vi "arrayMax.vi"(11 "Array":dbl[](array[numeric])) -> (3 "Maxed array":dbl[](array[numeric]))   [LabVIEW 2012]
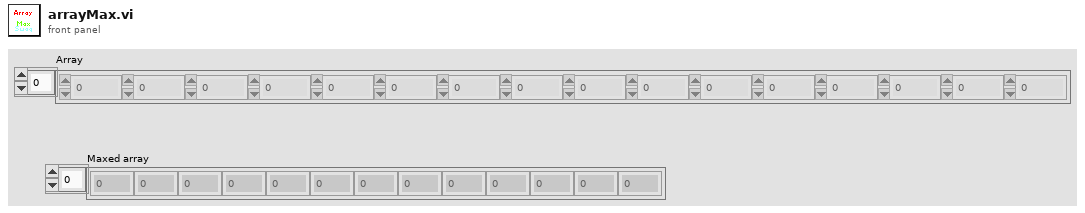
[diagram p1: front panel]
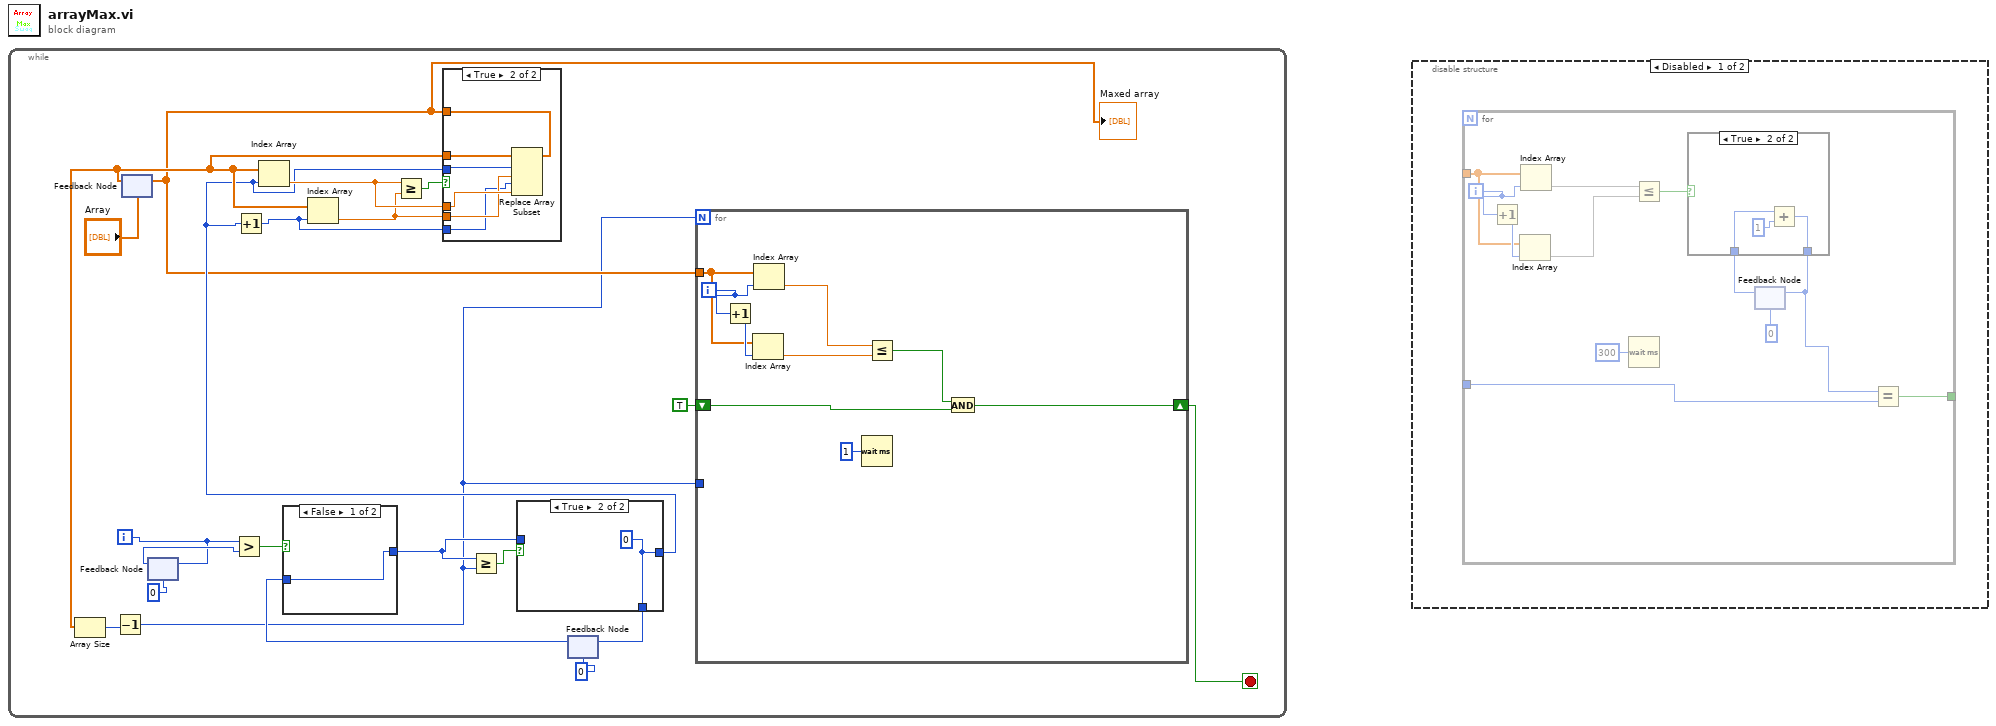
[diagram p0: block diagram]
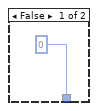
[diagram p2: hidden frame]
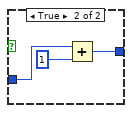
[diagram p5: hidden frame]
diagram:
  n1 = while {
    i -> [w18]
    stop <- w1 stop-if-true
    n2 = feedback #1("Array") -> (w10:dbl[])
    n3 = Array Size(array=w10) -> (size(s)=w4:i32)
    n4 = Decrement(x=w4) -> (x-1=w3:i32)
    n5 = feedback-in #2(w18) -> ()
    n6 = feedback #2(0) -> (w19:i32)
    n7 = Greater?(x=w18, y=w19) -> (0:w17:bool)
    n8 = feedback #3(0) -> (w8:i32)
    n9 = case shown="False" w17 {
      tunnel: [w33 w36] -> w15
      tunnel: w8 -> [w33 w34]
      frame False {
      }
      frame True {
        n10 = Add(x=w34, y=1) -> (x+y=w36:i32)
      }
    }
    n11 = Greater Or Equal?(x=w15, y=w3) -> (x >= y?=w16:bool)
    n12 = case shown="True" w16 {
      tunnel: [w31 w32] -> w6
      tunnel: w15 -> [w31 _]
      tunnel: [w31 w32] -> w7
      frame False {
      }
      frame True {
        w32 = 0
      }
    }
    n13 = Increment(x=w6) -> (x+1=w14:i32)
    n14 = Index Array(array=w10, index=w6) -> (element=w13:dbl)
    n15 = Index Array(array=w10, index=w14) -> (element=w12:dbl)
    n16 = Greater Or Equal?(x=w13, y=w12) -> (x >= y?=w21:bool)
    n17 = case shown="True" w21 {
      tunnel: w10 -> [w37 w43]
      tunnel: w6 -> [_ w39]
      tunnel: w14 -> [_ w38]
      tunnel: w13 -> [_ w42]
      tunnel: w12 -> [_ w41]
      tunnel: [w37 w40] -> w5
      frame False {
      }
      frame True {
        n18 = Replace Array Subset(array=w43, new element #1=w41, index #1=w39, new element #2=w42, index #2=w38) -> (w40:dbl[])
      }
    }
    "Maxed array" <- w5
    n19 = feedback-in #1(w5) -> ()
    n20 = feedback-in #3(w7) -> ()
    n21 = for {
      N: w3 -> [_]
      tunnel: w5 -> [w27]
      tunnel: w3 -> [_]
      shift-right: [w22] -> w1
      shift-left: TRUE -> [w23]
      i -> [w26]
      n22 = Increment(x=w26) -> (x+1=w30:i32)
      n23 = Index Array(array=w27, index=w30) -> (element=w28:dbl)
      n24 = Index Array(array=w27, index=w26) -> (element=w29:dbl)
      n25 = Wait (ms)(milliseconds to wait=u32 1) -> ()  [unwired: 1 out]
      n26 = Less Or Equal?(x=w29, y=w28) -> (x <= y?=w24:bool)
      n27 = And(x=w24, y=w23) -> (x .and. y?=w22:bool)
    }
  }
  n28 = disable-structure shown="Disabled" {
    frame Disabled {
      n29 = for {
        tunnel: _ -> [w51]
        tunnel: _ -> [w46]
        tunnel: [w47] -> _
        i -> [w45]
        n30 = Increment(x=w45) -> (x+1=w55:i32)
        n31 = Index Array(array=w51, index=w55) -> (element=w52)
        n32 = Index Array(array=w51, index=w45) -> (element=w53)
        n33 = Wait (ms)(milliseconds to wait=u32 300) -> ()  [unwired: 1 out]
        n34 = Less Or Equal?(x=w53, y=w52) -> (x <= y?=w54:bool)
        n35 = feedback #4(0) -> (w49:i32)
        n36 = case shown="True" w54 {
          tunnel: [0 w58] -> w48
          tunnel: w49 -> [_ w57]
          frame False {
          }
          frame True {
            n37 = Add(x=w57, y=1) -> (x+y=w58:i32)
          }
        }
        n38 = feedback-in #4(w48) -> ()
        n39 = Equal?(x=w48, y=w46) -> (x = y?=w47:bool)
      }
    }
    frame Enabled {
    }
  }
